vi "Analog Write.vi"(7 "Analog Ref Override":dbl, 8 "Error In":errorcluster={"status"=TRUE, "code"=5001, "source"="LVH-LINX.lvlib:Generate Error.vi<ERR>\nA timeout occured while waiting for the LINX device to respond."}, 9 "AO Values":dbl[](array[numeric]), 10 "AO Channels":u8[](array[numeric])=[0], 11 "LINX Device Config":T1={"Interface"=enum."Serial", "COM Port"="COM5", "TCP Configuration"={"IP Address"="", "Port"=0}, "Device Family"=0, "Device ID"=0, "Device Name"="", "TCP Ref"=refnum, "Channels"={"DI"=[], "DO"=[], "AI"=[], "AO"=[], "PWM"=[], "QE"=[], "UART"=[], "I2C 2"=[], "SPI"=[], "CAN"=[], "Servo"=[], "AI Ref (V)"=0.0, "AO Ref (V)"=0.0, "AO Resolution (Bits)"=0}}) -> (0 "Error Out":errorcluster={"status"=TRUE, "code"=5001, "source"="LVH-LINX.lvlib:Generate Error.vi<ERR>\nA timeout occured while waiting for the LINX device to respond."}, 3 "LINX Device Config":T1={"Interface"=enum."Serial", "COM Port"="COM5", "TCP Configuration"={"IP Address"="", "Port"=0}, "Device Family"=0, "Device ID"=0, "Device Name"="", "TCP Ref"=refnum, "Channels"={"DI"=[], "DO"=[], "AI"=[], "AO"=[], "PWM"=[], "QE"=[], "UART"=[], "I2C 2"=[], "SPI"=[], "CAN"=[], "Servo"=[], "AI Ref (V)"=0.0, "AO Ref (V)"=0.0, "AO Resolution (Bits)"=0}})   [LabVIEW 2011, in "LMH-LINX.lvlib" / "Device.lvlib"]
doc: "This VI Assumes a AO range of 0 to AREF"
uses:
  Device.lvlib
  Type Defs/LINX Device Config.ctl
  Type Defs/Interface.ctl
  Type Defs/TCP Config.ctl
  Type Defs/Channels.ctl
  Type Defs/Error Type.ctl
  LMH-LINX.lvlib
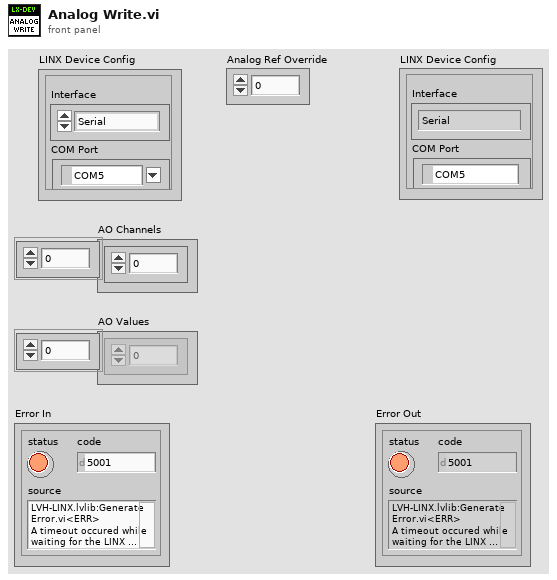
[diagram p1: front panel]
types:
  T1 = typedef "LMH-LINX.lvlib/Device.lvlib/LINX Device Config.ctl" = cluster{"Interface":T2, "COM Port":refnum<visa-resource-name>, "TCP Configuration":T3, "Device Family":u8, "Device ID":u8, "Device Name":string, "TCP Ref":refnum<k5>, "Channels":T4}
  T2 = typedef "LMH-LINX.lvlib/Interface.ctl" = enum16{"Serial", "TCP"}
  T3 = typedef "LMH-LINX.lvlib/Device.lvlib/TCP Config.ctl" = cluster{"IP Address":string, "Port":u16}
  T4 = typedef "LMH-LINX.lvlib/Channels.ctl" = cluster{"DI":u8[], "DO":u8[], "AI":u8[], "AO":u8[], "PWM":u8[], "QE":u8[], "UART":u8[], "I2C 2":u8[], "SPI":u8[], "CAN":u8[], "Servo":u8[], "AI Ref (V)":dbl, "AO Ref (V)":dbl, "AO Resolution (Bits)":u8}
  T5 = typedef "LMH-LINX.lvlib/Error Type.ctl" = enum16{"Unknown", "Timeout", "Corrupt Return Packet", "Unable To Connect", "Command Not Supported", "Channel DNE", "Invalid COM Config", "Firmware Version Mismatch", "myRIO Support", "CMD Specific Error"}
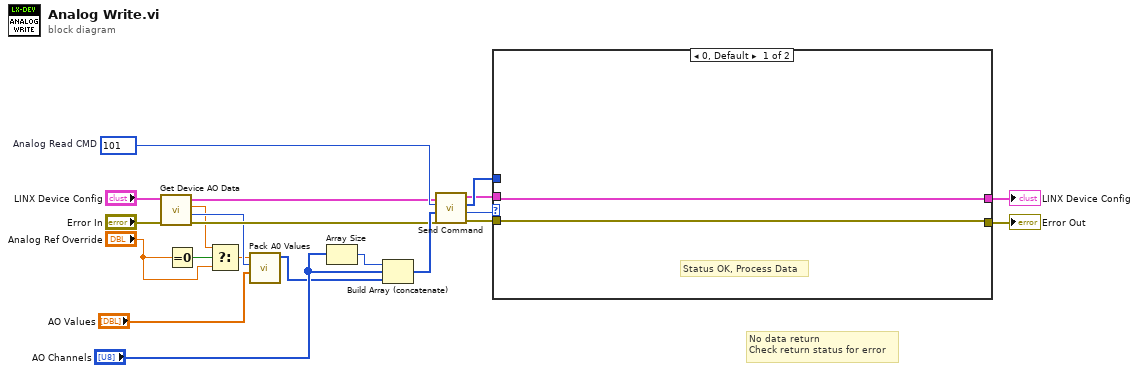
[diagram p0: block diagram]
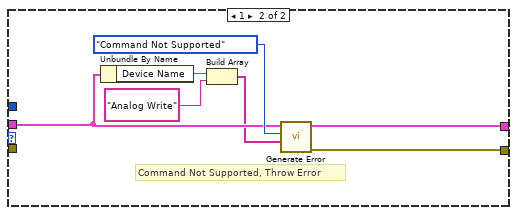
[diagram p2: hidden frame]
diagram:
  w21 = u16 101  # Analog Read CMD
  # "No data return\nCheck return status for error"
  n1 = call "Get Device AO Data.vi"("Error In"="Error In", "LINX Device Config"="LINX Device Config") -> ("Error Out"=w7:errorcluster, "AO Resolution (Bits)"=w5:u8, "AO Ref (V)"=w3:dbl, "LINX Device Config"=w11:T1)  [unwired: 6 in]
  n2 = Equal To 0?(x="Analog Ref Override") -> (x = 0?=w4:bool)
  n3 = Select(t=w3, s=w4, f="Analog Ref Override") -> (s? t:f=w1:dbl)
  n4 = call "Pack A0 Values.vi"("AO Values"="AO Values", "AO Resolution (Bits)"=w5, "Analog Ref Override"=w1) -> ("Packet Values"=w9:u8[])  [unwired: 8 in]
  n5 = Array Size(array="AO Channels") -> (size(s)=w16:i32)
  n6 = Build Array (concatenate)(w16, "AO Channels", w9) -> (w8:i32[])
  n7 = call "Send Command.vi"("Error In"=w7, "ARGS"=w8, "CMD"=w21, "LINX Device Config"=w11) -> ("Error Out"=w6:errorcluster, "Status"=w17:u8, "Response"=w18:u8[], "LINX Device Config"=w14:T1)  [unwired: 4 in]
  n8 = case shown="0, Default" w17 {
    tunnel: [w22 w29] -> w20
    tunnel: w14 -> [w22 w25]
    tunnel: [w23 w30] -> w19
    tunnel: w18 -> [_ _]
    tunnel: w6 -> [w23 _]
    frame 0, Default {
      # "Status OK, Process Data"
    }
    frame 1 {
      # "Command Not Supported, Throw Error"
      n9 = Unbundle By Name(w25) -> ("Device Name"=w27:string)
      n10 = Build Array(w27, "Analog Write") -> (w24:string[])
      n11 = call "Generate Error.vi"("Arguments"=w24, "Error Type"=Error_Type."Command Not Supported", "LINX Device Config"=w25) -> ("Error Out"=w30:errorcluster, "LINX Device Config"=w29:T1)  [unwired: 7 in]
    }
  }
  "Error Out" <- w19
  "LINX Device Config" <- w20
